vi "Configure Trigger (Holdoff).vi"(7 "Enable Random Trigger Mode (F: Disable)":bool, 8 "error in (no error)":errorcluster, 9 "Minimum Time (4E-8 S)":dbl=4e-08, 10 "Maximum Time (4.5E-8 S)":dbl=4.5e-08, 11 "VISA resource name":refnum<visa-resource-name>) -> (0 "error out":errorcluster, 3 "VISA resource name out":refnum<visa-resource-name>)   [LabVIEW 2017, in "Agilent 2000 3000 X-Series.lvlib"]
doc: "Configures the trigger holdoff mode. \n\n<b>Note:</b>\nThis VI is only applicable for 3000T, 4000, 6000 X-Series."
uses:
  Agilent 2000 3000 X-Series.lvlib
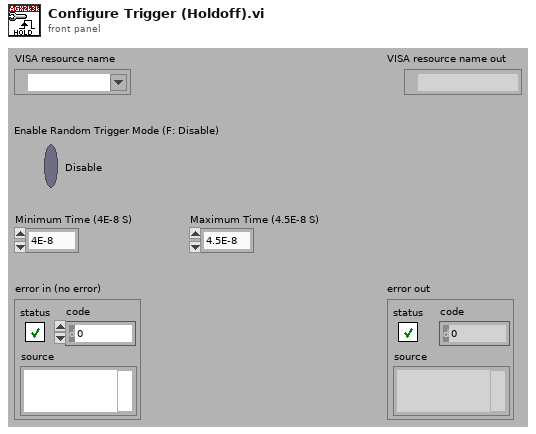
[diagram p1: front panel]
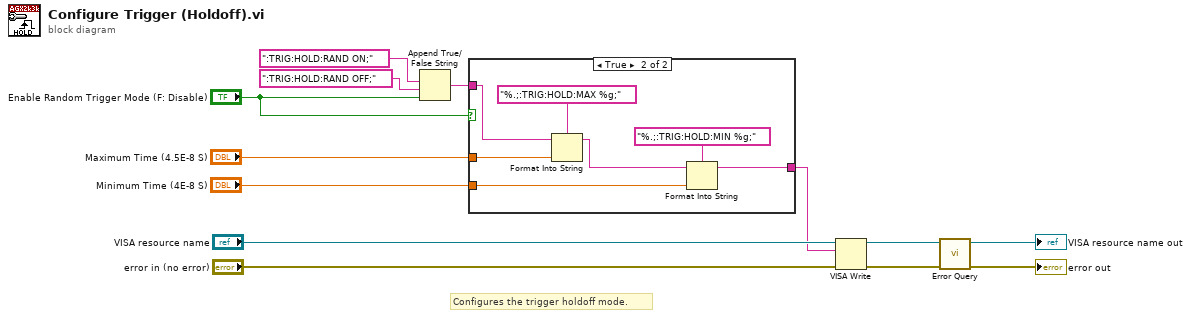
[diagram p0: block diagram]
diagram:
  # "Configures the trigger holdoff mode."
  n1 = Append True/False String(1:"Enable Random Trigger Mode (F: Disable)", 2:":TRIG:HOLD:RAND OFF;", 3:":TRIG:HOLD:RAND ON;") -> (0:w8:string)  [unwired: 1 in]
  n2 = case shown="True" "Enable Random Trigger Mode (F: Disable)" {
    tunnel: w8 -> [w14 w21]
    tunnel: "Maximum Time (4.5E-8 S)" -> [_ w20]
    tunnel: "Minimum Time (4E-8 S)" -> [_ w19]
    tunnel: [w14 w15] -> w1
    frame False {
    }
    frame True {
      n3 = Format Into String(format string="%.;:TRIG:HOLD:MAX %g;", initial string=w21, w20) -> (resulting string=w16:string)  [unwired: 1 in, 1 out]
      n4 = Format Into String(format string="%.;:TRIG:HOLD:MIN %g;", initial string=w16, w19) -> (resulting string=w15:string)  [unwired: 1 in, 1 out]
    }
  }
  n5 = VISA Write(VISA resource name="VISA resource name", write buffer=w1, error in (no error)="error in (no error)") -> (VISA resource name out=w5:refnum<visa-resource-name>, error out=w4:errorcluster)  [unwired: 1 out]
  n6 = call "Error Query.vi"("error in (no error)"=w4, "VISA resource name"=w5) -> ("error out"=→"error out":errorcluster, "VISA resource name out"=→"VISA resource name out":refnum<visa-resource-name>)  [unwired: 6 in, 2 out]
